vi "Get UI Details.vi"() -> ()   [LabVIEW 2021, in "DAQmxMeasurement1.lvlib"]
uses:
  DAQmxMeasurement1.lvlib
  <vilib>/Plug-In SDKs/Measurements/Helpers/TypeDefs/User Interface Information.ctl
  <vilib>/Plug-In SDKs/Measurements/NI Measurement Plug-In SDK.lvlib
panel:
  out "error out":errorcluster
  in  "error in":errorcluster
  out "user interface details":T1[](array[typedef])
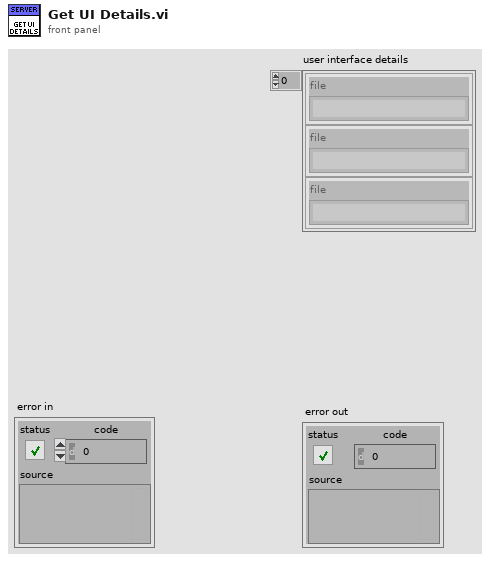
[diagram p1: front panel]
types:
  T1 = typedef "NI Measurement Plug-In SDK.lvlib/User Interface Information.ctl" = cluster{"file":string}
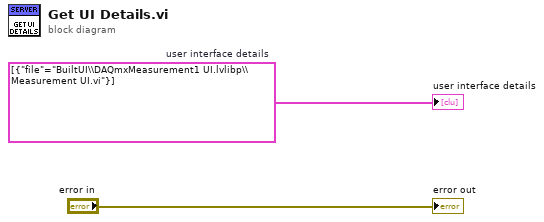
[diagram p0: block diagram]
diagram:
  w2 = T1[] [{"file"="BuiltUI\\DAQmxMeasurement1 UI.lvlibp\\Measurement UI.vi"}]  # user interface details
  "user interface details" <- w2
  "error out" <- "error in"
